vi "Get_Latest_Experiment_Settings.vi"(8 "error in (no error)":errorcluster, 11 "Small?":bool) -> (0 "error out":errorcluster, 1 "Experiment":string[](array[string]), 2 "Group":string, 3 "Integer Timestamp":dbl)   [LabVIEW 2013]
uses:
  <vilib>/addons/database/Connection.llb/Conn Execute.vi
  <vilib>/addons/database/Recordset.llb/Rec Fetch Recordset Data (R).vi
  <vilib>/addons/database/Recordset.llb/Rec Destroy - Connection.vi
  <vilib>/addons/database/_DB Variant To Data/Database Variant To Data.xnode
  <vilib>/addons/database/NI_Database_API.lvlib
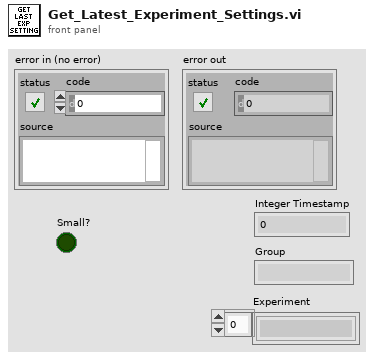
[diagram p1: front panel]
types:
  T1 = typedef "NI_Database_API.lvlib/Conn ObjectReference.ctl" = refnum<k1>
  T2 = typedef "NI_Database_API.lvlib/Rec ObjectReference.ctl" = refnum<k1>
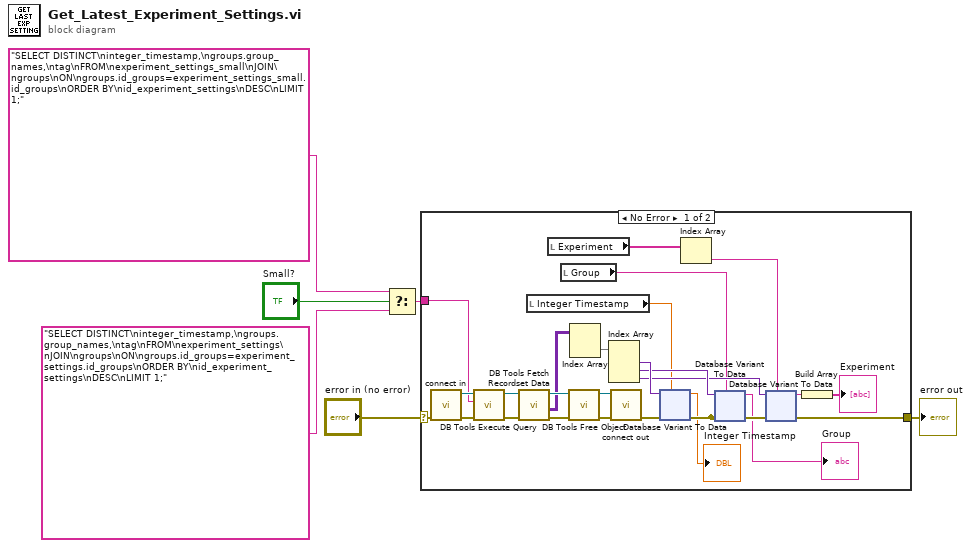
[diagram p0: block diagram]
diagram:
  n1 = Select(t="SELECT DISTINCT\ninteger_timestamp,\ngroups.group_names,\ntag\nFROM\nexperiment_settings_small\nJOIN\ngroups\nON\ngroups.id_groups=experiment_settings_small.id_groups\nORDER BY\nid_experiment_settings\nDESC\nLIMIT 1;" ("format string"), s="Small?", f="SELECT DISTINCT\ninteger_timestamp,\ngroups.group_names,\ntag\nFROM\nexperiment_settings\nJOIN\ngroups\nON\ngroups.id_groups=experiment_settings.id_groups\nORDER BY\nid_experiment_settings\nDESC\nLIMIT 1;" ("format string")) -> (s? t:f=w3:string)
  n2 = case shown="No Error" "error in (no error)" {
    selector: "error in (no error)" -> [w8 w129]
    tunnel: [w20 w129] -> w5
    tunnel: w3 -> [w7 _]
    frame No Error {
      n3 = call "connect in.vi"("error in (no error)"=w8) -> ("error out"=w31:errorcluster, "Database Connection"=w30:T1)  [unwired: 6 in, 1 out]
      n4 = call-poly <vilib>:"DB Tools Execute Query.vi"("error in (no error)"=w31, "SQL query"=w7, "connection reference"=w30) -> ("error out"=w29:errorcluster, "recordset reference"=w28:T2)  [unwired: 5 in]
      n5 = call-poly <vilib>:"DB Tools Fetch Recordset Data.vi"("error in (no error)"=w29, "recordset reference"=w28) -> ("error out"=w27:errorcluster, "recordset data"=w23:variant[][], "recordset reference out"=w32:T2)  [unwired: 3 in]
      n6 = local read "Integer Timestamp"() -> (w16:dbl)
      n7 = local read "Experiment"() -> (w14:string[])
      n8 = local read "Group"() -> (w15:string)
      n9 = call-poly <vilib>:"DB Tools Free Object.vi"("error in (no error)"=w27, "recordset reference"=w32) -> ("error out"=w25:errorcluster, "connection reference"=w26:T1)  [unwired: 8 in]
      n10 = Index Array(array=w23) -> (element=w22:variant[])  [unwired: 2 in]
      n11 = Index Array(array=w22) -> (element #1=w21:variant, element #2=w18:variant, element #3=w17:variant)  [unwired: 3 in]
      n12 = call "connect out.vi"("error in (no error)"=w25, "connection reference"=w26) -> ("error out"=w24:errorcluster)  [unwired: 9 in]
      n13 = xnode "Database Variant To Data"("database variant"=w21, "error in (no error)"=w24, "type"=w16) -> ("data"=→"Integer Timestamp":dbl, "error out"=w20:errorcluster)
      n14 = Index Array(array=w14) -> (element=w13:string)  [unwired: 1 in]
      n15 = xnode "Database Variant To Data"("database variant"=w18, "error in (no error)"=w20, "type"=w15) -> ("data"=→"Group":string, "error out"=w19:errorcluster)
      n16 = xnode "Database Variant To Data"("database variant"=w17, "error in (no error)"=w19, "type"=w13) -> ("data"=w10:string)  [unwired: 1 out]
      n17 = Build Array(w10) -> (→"Experiment":string[])
    }
    frame Error {
    }
  }
  "error out" <- w5
